vi "Read Full Module Name.vi"(8 "error in (no error)":errorcluster, 11 "JSON Routing Channel Template in":refnum<class "JSON Routing Channel Template.lvclass">) -> (0 "error out":errorcluster, 2 "Full Module Name":string, 3 "JSON Routing Channel Template out":refnum<class "JSON Routing Channel Template.lvclass">)   [LabVIEW 2020, in "Routing Templates.lvlib" / "JSON Routing Channel Template.lvclass"]
uses:
  JSON Routing Channel Template.lvclass
  JSON Routing Channel Template.lvclass/JSON Routing Channel Template.ctl
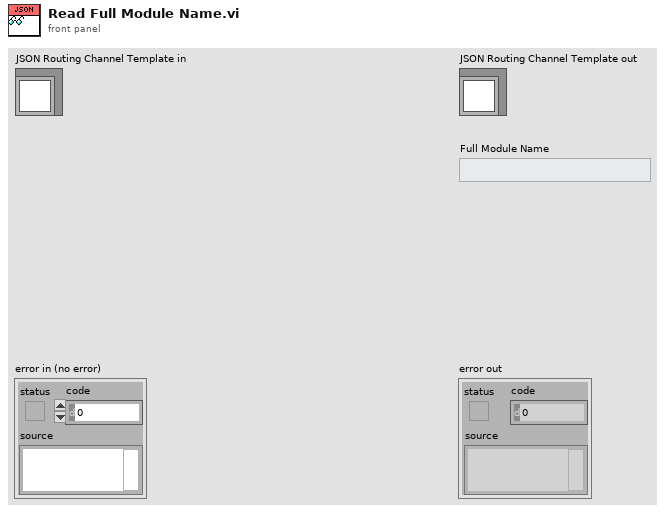
[diagram p1: front panel]
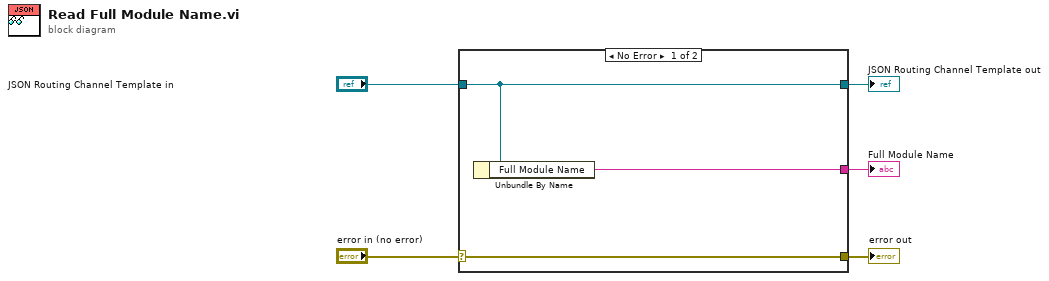
[diagram p0: block diagram]
diagram:
  n1 = case shown="No Error" "error in (no error)" {
    selector: "error in (no error)" -> [w8 w9]
    tunnel: [w8 w9] -> w4
    tunnel: [w7 w10] -> w2
    tunnel: "JSON Routing Channel Template in" -> [w7 w10]
    tunnel: [w6 _] -> w1
    frame No Error {
      n2 = Unbundle By Name(w7) -> ("Full Module Name"=w6:string)
    }
    frame Error {
    }
  }
  "error out" <- w4
  "JSON Routing Channel Template out" <- w2
  "Full Module Name" <- w1
